vi "G4BaseTemplate_Singleton_6x8x6_GetAttributes.vi"(0 "reference in":refnum<class "G4BaseTemplate_Singleton_6x8x6.lvclass">, 1 "OnlyGetDvrReference(False)":bool, 5 "error in (no error)":errorcluster) -> (14 "reference out":refnum<class "G4BaseTemplate_Singleton_6x8x6.lvclass">, 15 "Data":T1, 17 "DataRef":refnum<data-value>, 19 "error out":errorcluster)   [LabVIEW 2020, in "G4BaseTemplate_Singleton_6x8x6.lvclass"]
uses:
  <resource>/Framework/Providers/Open_GDS/ClassProviders/Provider_EndevoGOOP400/Templates/G4BaseTemplate_Singleton_6x8x6/G4BaseTemplate_Singleton_6x8x6.lvclass
  <resource>/Framework/Providers/Open_GDS/ClassProviders/Provider_EndevoGOOP400/Templates/G4BaseTemplate_Singleton_6x8x6/protected/ObjectAttributes.ctl
  <resource>/Framework/Providers/Open_GDS/ClassProviders/Provider_EndevoGOOP400/Templates/G4BaseTemplate_Singleton_6x8x6/G4BaseTemplate_Singleton_6x8x6.lvclass/G4BaseTemplate_Singleton_6x8x6.ctl
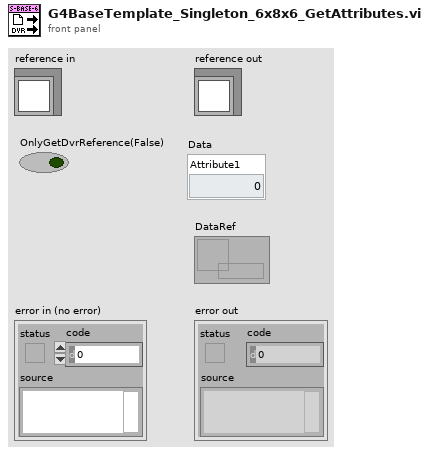
[diagram p1: front panel]
types:
  T1 = typedef "G4BaseTemplate_Singleton_6x8x6.lvclass/ObjectAttributes.ctl" = cluster{"Attribute1":dbl}
  T2 = typedef "G4BaseTemplate_Simple_6x8x6.lvclass/ObjectAttributes.ctl" = cluster{"Attribute1":dbl}
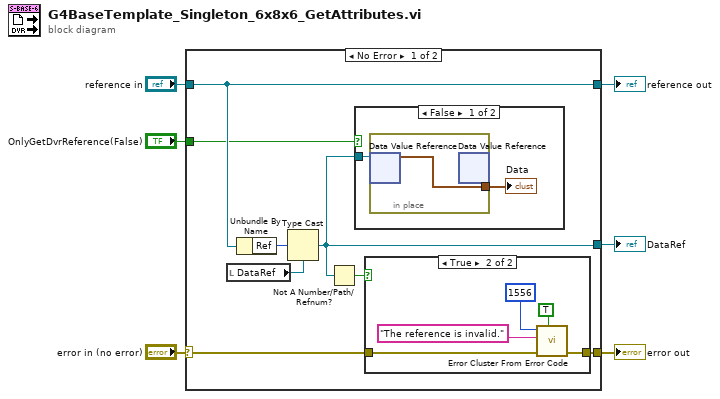
[diagram p0: block diagram]
diagram:
  n1 = case shown="No Error" "error in (no error)" {
    selector: "error in (no error)" -> [w8 w24]
    tunnel: [w7 w24] -> w5
    tunnel: [w14 w25] -> w3
    tunnel: "reference in" -> [w14 w25]
    tunnel: [w10 _] -> w2
    tunnel: "OnlyGetDvrReference(False)" -> [w11 _]
    frame No Error {
      n2 = local read "DataRef"() -> (w12:refnum<data-value>)
      n3 = Unbundle By Name(w14) -> ("Ref"=w13:u32)
      n4 = Type Cast(type=w12, x=w13) -> (*(type *) &x=w10:refnum<data-value>)
      n5 = Not A Number/Path/Refnum?(number/path/refnum=w10) -> (NaN/Path/Refnum?=w9:bool)
      n6 = case shown="False" w11 {
        tunnel: w10 -> [w22 _]
        frame False {
          n7 = in-place {
            in-place-border: [w23] -> w21
            n8 = in-place-dvr #1(w22) -> (w23:T2)  [unwired: 1 out]
            n9 = in-place-dvr #1() -> ()  [unwired: 1 in, 2 out]
          }
          "Data" <- w21
        }
        frame True {
        }
      }
      n10 = case shown="True" w9 {
        tunnel: w8 -> [w15 w17]
        tunnel: [w15 w16] -> w7
        frame False {
        }
        frame True {
          n11 = call <vilib>:"Error Cluster From Error Code.vi"("show call chain? (False)"=TRUE, "error in (no error)"=w17, "error message (\"\")"="The reference is invalid." ("source"), "error code (0)"=1556 ("code")) -> ("error out"=w16:errorcluster)  [unwired: 5 in]
        }
      }
    }
    frame Error {
    }
  }
  "error out" <- w5
  "reference out" <- w3
  "DataRef" <- w2
